vi "SUB_MaxVolumeNI.vi"(1 "Wave Volume":u32=60000, 2 "Speaker Volume":u32=60000 max=65535) -> ()   [LabVIEW 2011]
panel:
  out "Success":bool
  # "Range 0 - 65535"
  # "Range 0 - 65535"
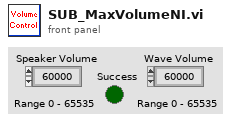
[diagram p1: front panel]
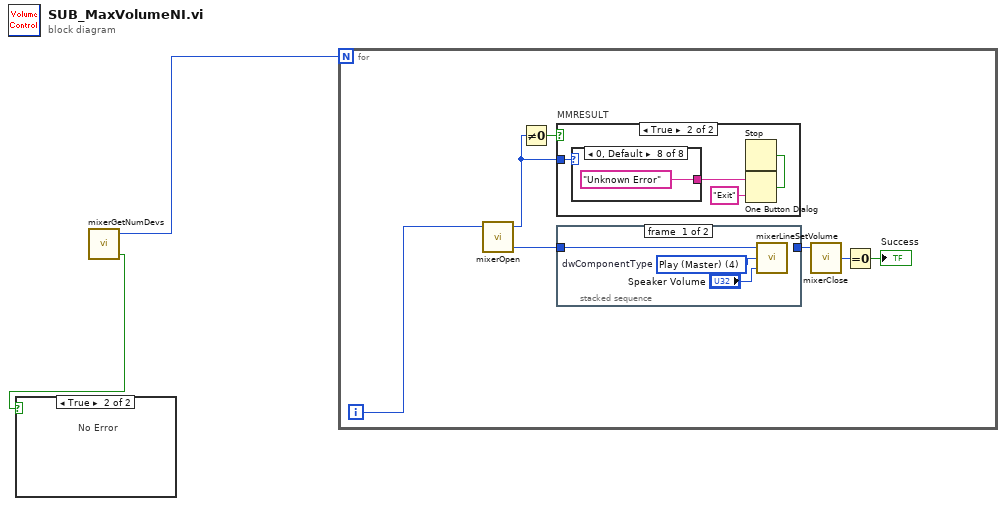
[diagram p0: block diagram]
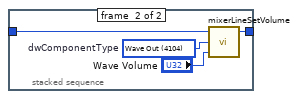
[diagram p2: hidden frame]
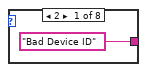
[diagram p4: hidden frame]
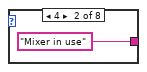
[diagram p5: hidden frame]
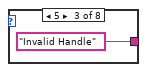
[diagram p6: hidden frame]
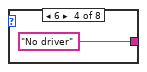
[diagram p7: hidden frame]
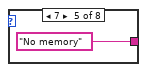
[diagram p8: hidden frame]
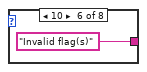
[diagram p9: hidden frame]
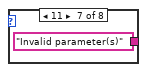
[diagram p10: hidden frame]
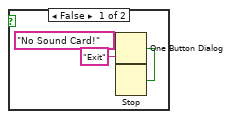
[diagram p11: hidden frame]
diagram:
  n1 = call "mixerGetNumDevs.vi"() -> ("Found"=w2:bool, "Number of\nMixer Devices"=w1:u32)  [unwired: 4 in]
  n2 = case shown="True" w2 {
    frame False {
      n3 = One Button Dialog(message="No Sound Card!", button name ("OK")="Exit") -> (true=w3:bool)
      n4 = Stop(stop? (T)=w3) -> ()
    }
    frame True {
      # "No Error"
    }
  }
  n5 = for {
    N: w1 -> [_]
    i -> [w6]
    n6 = call "mixerOpen.vi"("uMxId"=w6) -> ("phmx"=w10:u32, "MMRESULT"=w11:u32)  [unwired: 3 in]
    n7 = Not Equal To 0?(x=w11) -> (x != 0?=w12:bool)
    n8 = case "MMRESULT" shown="True" w12 {
      tunnel: w11 -> [_ w23]
      frame False {
        # "No Error"
      }
      frame True {
        n9 = case shown="0, Default" w23 {
          tunnel: ["Bad Device ID" ("message") "Mixer in use" ("message") "Invalid Handle" ("message") "No driver" ("message") "No memory" ("message") "Invalid flag(s)" ("message") "Invalid parameter(s)" ("message") "Unknown Error" ("message")] -> w21
          frame 2 {
          }
          frame 4 {
          }
          frame 5 {
          }
          frame 6 {
          }
          frame 7 {
          }
          frame 10 {
          }
          frame 11 {
          }
          frame 0, Default {
          }
        }
        n10 = One Button Dialog(message=w21, button name ("OK")="Exit") -> (true=w20:bool)
        n11 = Stop(stop? (T)=w20) -> ()
      }
    }
    n12 = stacked-sequence {
      tunnel: w10 -> [w14 w19]
      tunnel: [_ w16] -> w7
      frame #0 {
        w13 = u32 4 items=["Play (Master)"=4, "CD Audio"=4112, "Line In"=4098, "Microphone In"=4099, "PC Speaker"=4103, "Auxiliary In"=4105, "TAD In"=4102, "Wave Out"=4104, "MIDI"=4100, "CD Digital"=4097]  # dwComponentType
        n13 = call "mixerLineSetVolume.vi"("Volume"="Speaker Volume", "dwComponentType"=w13, "hmxobj"=w14) -> ()  [unwired: 1 in, 2 out]
      }
      frame #1 {
        w18 = u32 4104 items=["Play (Master)"=4, "CD Audio"=4112, "Line In"=4098, "Microphone In"=4099, "PC Speaker"=4103, "Auxiliary In"=4105, "TAD In"=4102, "Wave Out"=4104, "MIDI"=4100, "CD Digital"=4097]  # dwComponentType
        n14 = call "mixerLineSetVolume.vi"("Volume"="Wave Volume", "dwComponentType"=w18, "hmxobj"=w19) -> ("hmxobj Out"=w16:u32)  [unwired: 1 in, 1 out]
      }
    }
    n15 = call "mixerClose.vi"("hmx"=w7) -> ("MMRESULT"=w8:u32)  [unwired: 4 in]
    n16 = Equal To 0?(x=w8) -> (x = 0?=→"Success":bool)
  }
